vi "NI VeriStand - Get Item Data.vi"(8 "error in (no error)":errorcluster, 11 "Item Ref in":T2 format="%.0x") -> (0 "error out":errorcluster, 2 "Item Info":T1, 3 "Item Ref out":T2 format="%.0x", 4 "Found":bool)   [LabVIEW 2026, in "Custom Devices Storage.lvlib"]
uses:
  Custom Devices Storage.lvlib
  <vilib>/NI VeriStand/Custom Device API/Custom Device Item Ref.ctl
  <vilib>/NI VeriStand/Custom Device API/Custom Device Item Info.ctl
  C:/Users/Administrator/Desktop/Jatin/All DNC DLLs/NationalInstruments.VeriStand.SystemDefinitionAPI.dll
  Jatin/All DNC DLLs/NationalInstruments.VeriStand.SystemDefinitionAPI.dll
  C:/Users/Administrator/Desktop/Jatin/All DNC DLLs/NationalInstruments.VeriStand.SystemStorage.dll
  Jatin/All DNC DLLs/NationalInstruments.VeriStand.SystemStorage.dll
  <vilib>/NI VeriStand/Custom Device API/Custom Device API.lvlib
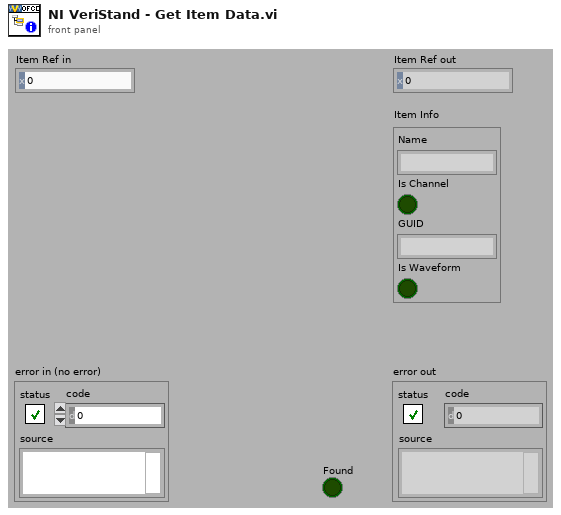
[diagram p1: front panel]
types:
  T1 = typedef "Custom Device API.lvlib/Custom Device Item Info.ctl" = cluster{"Name":string, "Is Channel":bool, "GUID":string, "Is Waveform":bool}
  T2 = typedef "Custom Device API.lvlib/Custom Device Item Ref.ctl" = u64
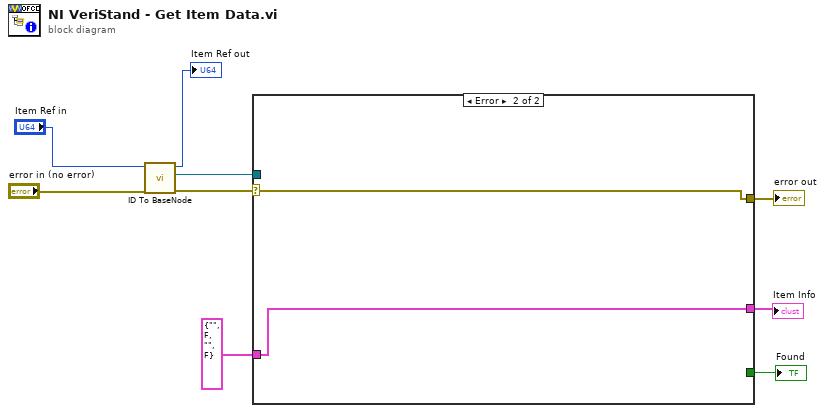
[diagram p0: block diagram]
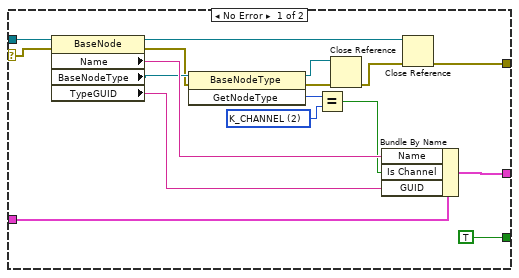
[diagram p2: hidden frame]
diagram:
  n1 = call "ID To BaseNode.vi"("error in (no error)"="error in (no error)", "ID in"="Item Ref in") -> ("error out"=w7:errorcluster, "NationalInstruments.VeriStand.SystemDefinitionAPI.BaseNode"=w6:refnum<k39>, "ID out"=→"Item Ref out":u64)  [unwired: 7 in]
  n2 = case shown="Error" w7 {
    selector: w7 -> [w26 w28]
    tunnel: w6 -> [w25 _]
    tunnel: T1 {"Name"="", "Is Channel"=FALSE, "GUID"="", "Is Waveform"=FALSE} ("Item Info") -> [w24 w27]
    tunnel: [w14 w27] -> w3
    tunnel: [w11 w28] -> w2
    tunnel: [TRUE _] -> w1
    frame No Error {
      w19 = 2 items=["K_BASE", "K_ALIAS", "K_CHANNEL", "K_SECTION", "K_TARGET", "K_TARGETSECTION", "K_ROOT"] ("GetNodeType")
      n3 = property class="BaseNode"(reference=w25, error in=w26) -> (reference out=w13:refnum<k39>, error out=w21:errorcluster, "Name"=w23:string, "BaseNodeType"=w22:refnum<k39>, "TypeGUID"=w15:string)
      n4 = invoke class="BaseNodeType" method="GetNodeType"(reference=w22, error in=w21) -> (reference out=w17:refnum<k39>, error out=w18:errorcluster, "GetNodeType"=w20:i32)  [unwired: 1 in]
      n5 = Equal?(x=w20, y=w19) -> (x = y?=w16:bool)
      n6 = Close Reference(reference=w17, error in (no error)=w18) -> (error out=w12:errorcluster)
      n7 = Bundle By Name(cluster=w24, "Name"=w23, "Is Channel"=w16, "GUID"=w15) -> (w14:T1)
      n8 = Close Reference(reference=w13, error in (no error)=w12) -> (error out=w11:errorcluster)
    }
    frame Error {
    }
  }
  "error out" <- w2
  "Found" <- w1
  "Item Info" <- w3
